vi "Header or Footer Close Ref.vi"(7 "Header or Footer Complete Cluster":T1, 11 "error in (no error)":errorcluster, 13 "Default Font":refnum<k24>) -> (15 "error out":errorcluster)   [LabVIEW 2012]
doc: "Version 1.0\nDeveloped by Jean-Marc Simard\nCopyright © 2010, Exaprom Inc.\nAll rights reserved.\nLicense: BSD\n\nWith iTextSharp 4.1.6 (http://itextsharp.sourceforge.net)\nunder Mozilla Public License Version 1.1\n(http://www.mozilla.org/MPL/MPL-1.1.html)"
uses:
  Controls/Header Footer Complete Cluster.ctl
  Controls/Header Footer Cluster with references.ctl
  Controls/Header Footer Type.ctl
  Controls/Header footer horiz alignment.ctl
  Controls/Cell Vertical alignment.ctl
  Controls/Page number.ctl
  C:/Users/MaxCorp/Documents/TopPerm - Base/DLL/itextsharp.dll
  DLL/itextsharp.dll
  Controls/Font cluster.ctl
  Controls/Font size.ctl
  Controls/Font color.ctl
  Controls/Header Footer Line.ctl
panel:
  # "X"
  # "Y"
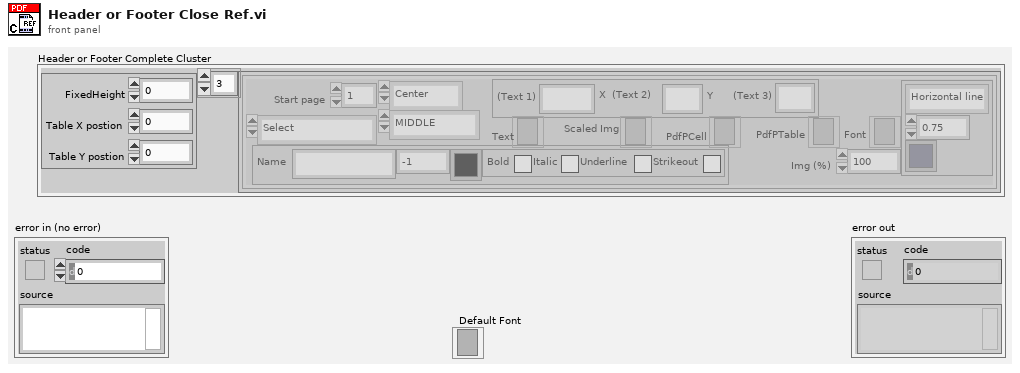
[diagram p1: front panel]
types:
  T1 = typedef "Header Footer Complete Cluster.ctl" = cluster{"Table position":cluster{"FixedHeight":dbl, "Table X postion":dbl, "Table Y postion":dbl}, "Header Footer Cluster with references [ ]":T2[]}
  T2 = typedef "Header Footer Cluster with references.ctl" = cluster{"Start page":i32, "Type":T3, "Alignment":T4, "Vertical Alignement":T5, "Page #":T6, "Text":refnum<k24>, "Scaled Img":refnum<k24>, "PdfPCell":refnum<k24>, "PdfPTable":refnum<k24>, "Font Cluster":T7, "Font ":refnum<k24>, "Img (%)":sgl, "Line":cluster{"Line":T10, "Thickness (points)":sgl, "Colour":T9}}
  T3 = typedef "Header Footer Type.ctl" = enum16{"Select", "Text", "Text + hyperlink", "Page number", "Image", "Image + hyperlink"}
  T4 = typedef "Header footer horiz alignment.ctl" = enum16{"Left", "Center", "Right"}
  T5 = typedef "Cell Vertical alignment.ctl" = enum16{"TOP", "MIDDLE", "BOTTOM"}
  T6 = typedef "Page number.ctl" = cluster{"Text 1":string, "Text 2":string, "Text 3":string}
  T7 = typedef "Font cluster.ctl" = cluster{"Name":string, "Size":T8, "Color":T9, "Style":cluster{"Bold":bool, "Italic":bool, "Underline":bool, "Strikeout":bool}}
  T8 = typedef "Font size.ctl" = sgl
  T9 = typedef "Font color.ctl" = u32
  T10 = typedef "Header Footer Line.ctl" = enum16{"No line", "Horizontal line"}
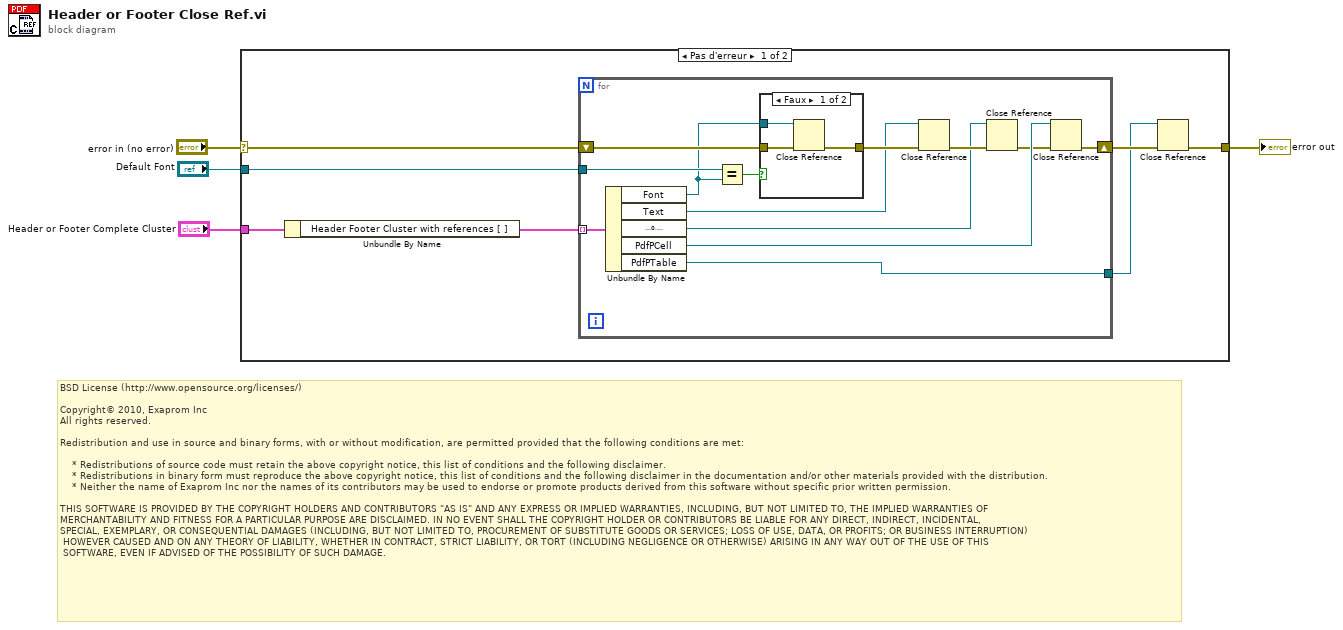
[diagram p0: block diagram]
diagram:
  # "BSD License (http://www.opensource.org/licenses/)\n\nCopyright© 2010, Exaprom Inc\nAll rights reserved.\n\nRedistribution and use in source and binary forms, with or without modification, are permitted provided that the following conditions are met:\n\n    * Redistributions of source code must retain the above copyright notice, this list of conditions and the following disclaimer.\n    * Redistributions in binary form must reproduce the above copyright notice, this list of conditions and the following disclaimer in the documentation and/or other materials provided with the distribution.\n    * Neither the name of Exaprom Inc nor the names of its contributors may be used to endorse or promote products derived from this software without specific prior written permission.\n\nTHIS SOFTWARE IS PROVIDED BY THE COPYRIGHT HOLDERS AND CONTRIBUTORS \"AS IS\" AND ANY EXPRESS OR IMPLIED WARRANTIES, INCLUDING, BUT NOT LIMITED TO, THE IMPLIED WARRANTIES OF \nMERCHANTABILITY AND FITNESS FOR A PARTICULAR PURPOSE ARE DISCLAIMED. IN NO EVENT SHALL THE COPYRIGHT HOLDER OR CONTRIBUTORS BE LIABLE FOR ANY DIRECT, INDIRECT, INCIDENTAL,\nSPECIAL, EXEMPLARY, OR CONSEQUENTIAL DAMAGES (INCLUDING, BUT NOT LIMITED TO, PROCUREMENT OF SUBSTITUTE GOODS OR SERVICES; LOSS OF USE, DATA, OR PROFITS; OR BUSINESS INTERRUPTION)\n HOWEVER CAUSED AND ON ANY THEORY OF LIABILITY, WHETHER IN CONTRACT, STRICT LIABILITY, OR TORT (INCLUDING NEGLIGENCE OR OTHERWISE) ARISING IN ANY WAY OUT OF THE USE OF THIS\n SOFTWARE, EVEN IF ADVISED OF THE POSSIBILITY OF SUCH DAMAGE."
  n1 = case shown="Pas d'erreur" "error in (no error)" {
    selector: "error in (no error)" -> [w9 w29]
    tunnel: [w7 w29] -> w4
    tunnel: "Header or Footer Complete Cluster" -> [w11 _]
    tunnel: "Default Font" -> [w5 _]
    frame No Error {
      n2 = Unbundle By Name(w11) -> ("Header Footer Cluster with references [ ]"=w10:T2[])
      n3 = for {
        tunnel: w10 -> [w19] mode=indexing
        shift-right: [w22] -> w8
        shift-left: w9 -> [w24]
        tunnel: [w18] -> w6
        tunnel: w5 -> [w13]
        n4 = Unbundle By Name(w19) -> ("Font"=w12:refnum<k24>, "Text"=w21:refnum<k24>, "Scaled Img"=w15:refnum<k24>, "PdfPCell"=w20:refnum<k24>, "PdfPTable"=w18:refnum<k24>)
        n5 = Equal?(x=w13, y=w12) -> (x = y?=w14:bool)
        n6 = case shown="Faux" w14 {
          tunnel: w24 -> [w27 w28]
          tunnel: [w26 w28] -> w23
          tunnel: w12 -> [w25 _]
          frame False {
            n7 = Close Reference(reference=w25, error in (no error)=w27) -> (error out=w26:errorcluster)
          }
          frame True {
          }
        }
        n8 = Close Reference(reference=w21, error in (no error)=w23) -> (error out=w16:errorcluster)
        n9 = Close Reference(reference=w15, error in (no error)=w16) -> (error out=w17:errorcluster)
        n10 = Close Reference(reference=w20, error in (no error)=w17) -> (error out=w22:errorcluster)
      }
      n11 = Close Reference(reference=w6, error in (no error)=w8) -> (error out=w7:errorcluster)
    }
    frame Error {
    }
  }
  "error out" <- w4
